vi "decodeBin.vi"(8 "error in (no error)":errorcluster, 10 "ByteArray":u8[](array[numeric])) -> (0 "error out":errorcluster, 1 "BinaryArray":u8[](array[numeric]), 2 "variant":variant, 3 "RemainingBytes":u8[](array[numeric]), 5 "Type":string)   [LabVIEW 2016, in "MsgPack.lvlib"]
uses:
  MsgPack.lvlib
  <vilib>/Utility/error.llb/Error Cluster From Error Code.vi
  <vilib>/ErrorRing/Error Ring.xnode
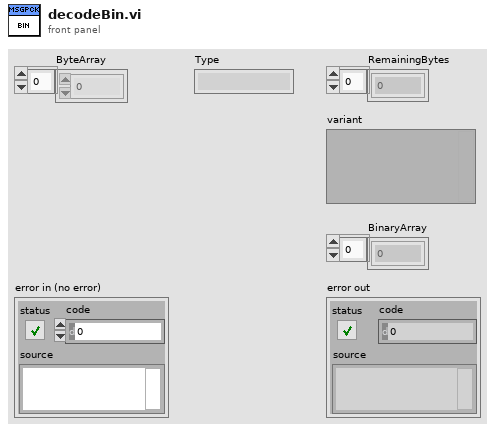
[diagram p1: front panel]
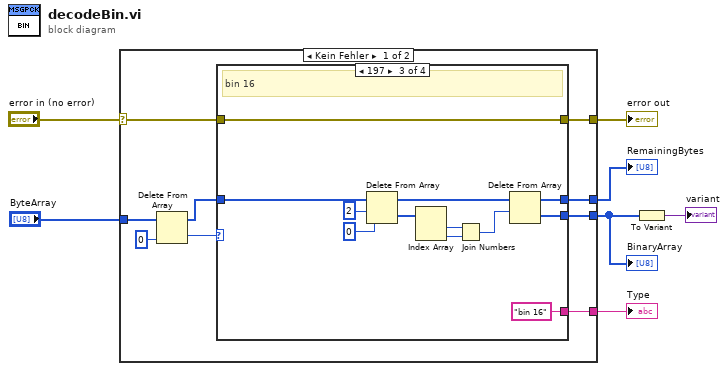
[diagram p0: block diagram]
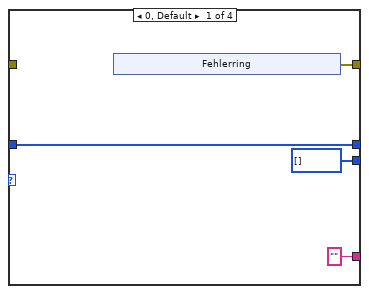
[diagram p2: hidden frame]
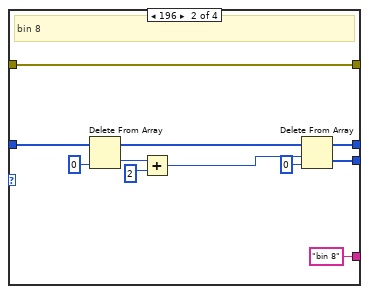
[diagram p3: hidden frame]
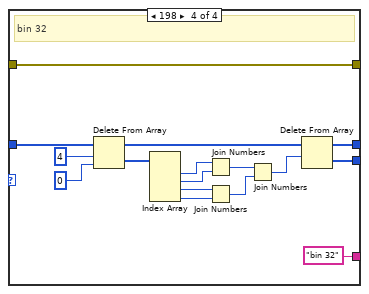
[diagram p4: hidden frame]
diagram:
  n1 = case shown="Kein Fehler" "error in (no error)" {
    selector: "error in (no error)" -> [w8 w66]
    tunnel: [w16 w66] -> w6
    tunnel: [w15 _] -> w5
    tunnel: [w14 _] -> w4
    tunnel: [w13 w65] -> w3
    tunnel: "ByteArray" -> [w12 w65]
    frame No Error {
      n2 = Delete From Array(array=w12, index=0) -> (deleted portion=w9:u8, array with subset deleted=w11:u8[])  [unwired: 1 in]
      n3 = case shown="197" w9 {
        tunnel: [w19 w34 w47 w63] -> w16
        tunnel: w8 -> [_ w34 w47 w63]
        tunnel: ["" "bin 8" "bin 16" "bin 32"] -> w15
        tunnel: [u8[] [] w31 w39 w51] -> w14
        tunnel: w11 -> [w17 w28 w42 w56]
        tunnel: [w17 w32 w38 w50] -> w13
        frame 0, Default {
          n4 = xnode "Fehlerring"() -> ("Fehler (Ausgang)"=w19:errorcluster)
        }
        frame 196 {
          # "bin 8"
          n5 = Delete From Array(array=w28, index=0) -> (deleted portion=w27:u8, array with subset deleted=w26:u8[])  [unwired: 1 in]
          n6 = Add(x=w27, y=u8 2) -> (x+y=w33:u8)
          n7 = Delete From Array(array=w26, length=w33, index=0) -> (deleted portion=w31:u8[], array with subset deleted=w32:u8[])
        }
        frame 197 {
          # "bin 16"
          n8 = Delete From Array(array=w42, length=2, index=0) -> (deleted portion=w43:u8[], array with subset deleted=w41:u8[])
          n9 = Index Array(array=w43) -> (element #1=w45:u8, element #2=w46:u8)  [unwired: 2 in]
          n10 = Join Numbers(hi=w45, lo=w46) -> ((hi.lo)=w40:u16)
          n11 = Delete From Array(array=w41, length=w40) -> (deleted portion=w39:u8[], array with subset deleted=w38:u8[])  [unwired: 1 in]
        }
        frame 198 {
          # "bin 32"
          n12 = Delete From Array(array=w56, length=4, index=0) -> (deleted portion=w54:u8[], array with subset deleted=w53:u8[])
          n13 = Index Array(array=w54) -> (element #1=w61:u8, element #2=w62:u8, element #3=w60:u8, element #4=w59:u8)  [unwired: 4 in]
          n14 = Join Numbers(hi=w61, lo=w62) -> ((hi.lo)=w57:u16)
          n15 = Join Numbers(hi=w60, lo=w59) -> ((hi.lo)=w58:u16)
          n16 = Join Numbers(hi=w57, lo=w58) -> ((hi.lo)=w52:u32)
          n17 = Delete From Array(array=w53, length=w52) -> (deleted portion=w51:u8[], array with subset deleted=w50:u8[])  [unwired: 1 in]
        }
      }
    }
    frame Error {
    }
  }
  "error out" <- w6
  "Type" <- w5
  "BinaryArray" <- w4
  "RemainingBytes" <- w3
  n18 = To Variant(anything=w4) -> (Variant=→"variant":variant)
